vi "Acquire.vi"(8 "error in (no error)":errorcluster, 10 "Data Notifier":refnum<notifier>, 11 "Hardware Resources in":T1) -> (0 "error out":errorcluster, 3 "Hardware Resources out":T1)   [LabVIEW 2017, in "Acquisition.lvlib"]
doc: "Perform the acquisition. Replace the contents of this diagram with calls to acquisition hardware."
uses:
  Acquisition.lvlib
  Hardware Configuration.ctl
  <vilib>/DAQmx/read.llb/DAQmx Read (Analog 1D Wfm NChan NSamp).vi
  <vilib>/DAQmx/miscellaneous.llb/DAQmx Fill In Error Info.vi
  <resource>/objmgr/daqmx.rc
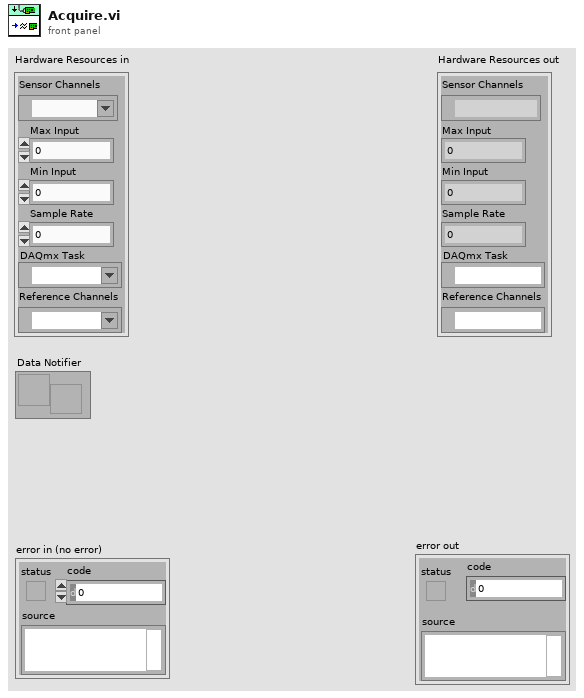
[diagram p1: front panel]
types:
  T1 = typedef "Acquisition.lvlib/Hardware Configuration.ctl" = cluster{"Sensor Channels":tag, "Max Input":dbl, "Min Input":dbl, "Sample Rate":dbl, "DAQmx Task":refnum<k21>, "Reference Channels":tag}
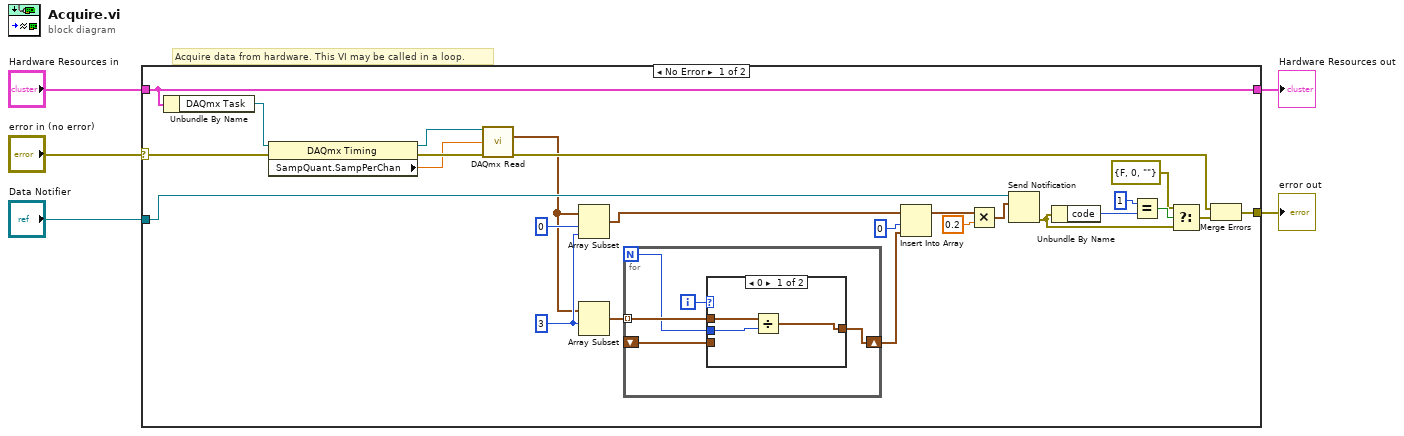
[diagram p0: block diagram]
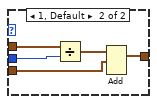
[diagram p2: hidden frame]
diagram:
  # "Acquire data from hardware. This VI may be called in a loop."
  n1 = case shown="No Error" "error in (no error)" {
    selector: "error in (no error)" -> [w18 w44]
    tunnel: [w30 w44] -> w4
    tunnel: "Hardware Resources in" -> [w22 w45]
    tunnel: [w22 w45] -> w2
    tunnel: "Data Notifier" -> [w29 _]
    frame No Error {
      w12 = 3 ("index")
      n2 = Unbundle By Name(w22) -> ("DAQmx Task"=w20:refnum<k21>)
      n3 = property class="DAQmx Timing"(reference=w20, error in=w18) -> (reference out=w19:refnum<k21>, error out=w17:errorcluster, "SampQuant.SampPerChan"=w16:dbl)
      n4 = call-poly <vilib>:"DAQmx Read.vi"("task/channels in"=w19, "number of samples per channel"=w16, "error in"=w17) -> ("data"=w10:waveform(dbl)[], "error out"=w21:errorcluster)  [unwired: 10 in, 1 out]
      n5 = Array Subset(array=w10, index=0, length=w12) -> (w9:waveform(dbl)[])
      n6 = Array Subset(array=w10, index=w12) -> (w13:waveform(dbl)[])  [unwired: 1 in]
      n7 = for {
        N -> [w33]
        tunnel: w13 -> [w35] mode=indexing
        shift-right: [w32] -> w8
        shift-left: _ -> [w31]
        i -> [w34]
        n8 = case shown="0" w34 {
          tunnel: w35 -> [w38 w42]
          tunnel: [w36 w41] -> w32
          tunnel: w33 -> [w37 w40]
          tunnel: w31 -> [_ w39]
          frame 0 {
            n9 = Divide(x=w38, y=w37) -> (x/y=w36:waveform(dbl))
          }
          frame 1, Default {
            n10 = Divide(x=w42, y=w40) -> (x/y=w43:waveform(dbl))
            n11 = Add(1:w39, 2:w43) -> (0:w41:waveform(dbl))  [unwired: 1 in, 1 out]
          }
        }
      }
      n12 = Insert Into Array(array=w9, index=0, new element=w8) -> (w15:waveform(dbl)[])
      n13 = Multiply(x=w15, y=0.2) -> (x*y=w7:waveform(dbl)[])
      n14 = Send Notification(notification=w7, notifier=w29) -> (error out=w25:errorcluster)  [unwired: 1 in, 1 out]
      n15 = Unbundle By Name(w25) -> ("code"=w28:i32)
      n16 = Equal?(x=1, y=w28) -> (x = y?=w26:bool)
      n17 = Select(t=errorcluster {"status"=FALSE, "code"=0, "source"=""} ("error constant"), s=w26, f=w25) -> (s? t:f=w24:errorcluster)
      n18 = Merge Errors(w21, w24) -> (w30:errorcluster)
    }
    frame Error {
    }
  }
  "Hardware Resources out" <- w2
  "error out" <- w4
